vi "Initialize Settings 1.0.vi"(8 "error in (no error)":errorcluster, 11 "settings 1.0":cluster{"key":string, "value":string}[](array[cluster])) -> (0 "error out":errorcluster, 3 "configuration 1.0":T1)   [LabVIEW 2021, in "DSF Core.lvlib" / "Plugin Configuration.lvclass"]
uses:
  Plugin Configuration.lvclass
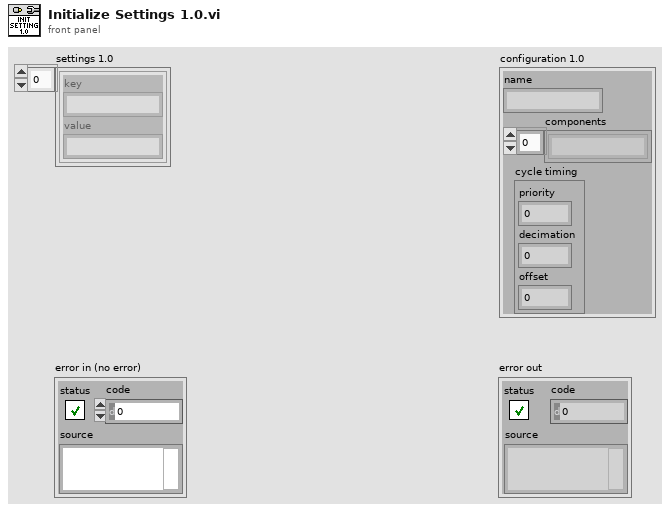
[diagram p1: front panel]
types:
  T1 = cluster{"name":string, "components":string[], "cycle timing":cluster{"priority":u64, "decimation":u64, "offset":u64}}
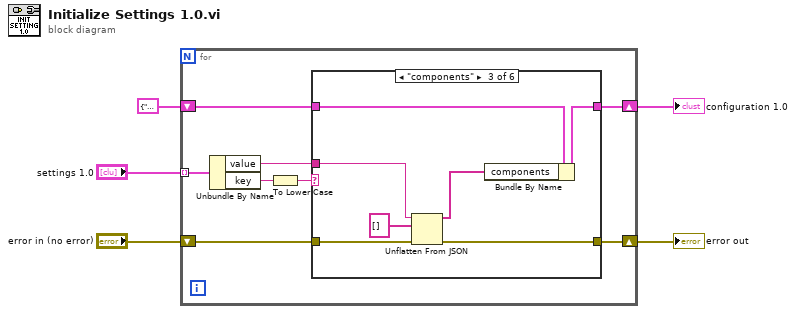
[diagram p0: block diagram]
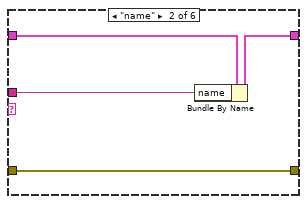
[diagram p3: hidden frame]
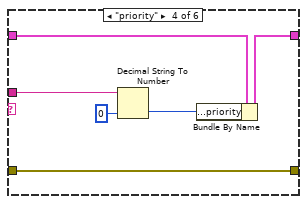
[diagram p4: hidden frame]
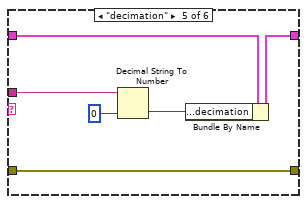
[diagram p5: hidden frame]
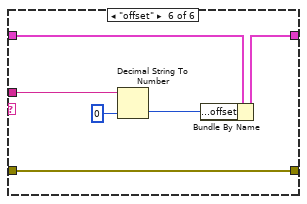
[diagram p6: hidden frame]
diagram:
  n1 = for {
    shift-right: [w8] -> w4
    shift-left: T1 {"name"="", "components"=[], "cycle timing"={"priority"=10000, "decimation"=1, "offset"=0}} ("configuration") -> [w9]
    tunnel: "settings 1.0" -> [w13] mode=indexing
    shift-right: [w6] -> w3
    shift-left: "error in (no error)" -> [w7]
    n2 = Unbundle By Name(w13) -> ("value"=w10:string, "key"=w12:string)
    n3 = To Lower Case(string=w12) -> (all lower case string=w11:string)
    n4 = case shown="\"components\"" w11 {
      tunnel: w10 -> [_ w17 w22 w28 w34 w40]
      tunnel: w9 -> [w15 w19 w26 w32 w38 w44]
      tunnel: [w15 w18 w25 w31 w37 w43] -> w8
      tunnel: w7 -> [w14 w16 w24 w30 w36 w42]
      tunnel: [w14 w16 w21 w30 w36 w42] -> w6
      frame Default {
        # "Unknown setting."
      }
      frame "name" {
        n5 = Bundle By Name(cluster=w19, "name"=w17) -> (w18:T1)
      }
      frame "components" {
        n6 = Unflatten From JSON(JSON string=w22, type and defaults=string[] [] ("components"), error in (no error)=w24) -> (value=w20:string[], error out=w21:errorcluster)  [unwired: 4 in]
        n7 = Bundle By Name(cluster=w26, "components"=w20) -> (w25:T1)
      }
      frame "priority" {
        n8 = Decimal String To Number(string=w28, default (0L)=u64 0 ("default (0 I32)")) -> (number=w29:u64)  [unwired: 1 in, 1 out]
        n9 = Bundle By Name(cluster=w32, "cycle timing.priority"=w29) -> (w31:T1)
      }
      frame "decimation" {
        n10 = Decimal String To Number(string=w34, default (0L)=u64 0 ("default (0 I32)")) -> (number=w35:u64)  [unwired: 1 in, 1 out]
        n11 = Bundle By Name(cluster=w38, "cycle timing.decimation"=w35) -> (w37:T1)
      }
      frame "offset" {
        n12 = Decimal String To Number(string=w40, default (0L)=u64 0 ("default (0 I32)")) -> (number=w41:u64)  [unwired: 1 in, 1 out]
        n13 = Bundle By Name(cluster=w44, "cycle timing.offset"=w41) -> (w43:T1)
      }
    }
  }
  "error out" <- w3
  "configuration 1.0" <- w4
